vi "ObjectHandler.GetSegmentRefsForCycle.vi"(8 "error in (no error)":errorcluster, 10 "CycleName":string, 11 "ObjectHandler in":refnum<class "ObjectHandler.lvclass">) -> (0 "error out":errorcluster, 2 "ObjectArray":T1[](array[typedef]), 3 "ObjectHandler out":refnum<class "ObjectHandler.lvclass">)   [LabVIEW 2016, in "ObjectHandler.lvclass"]
uses:
  ObjectHandler.lvclass
  ObjectHandler.ObjectWType.ctl
  ObjectHandler.ObjectType.ctl
  ObjectHandler.lvclass/ObjectHandler.ctl
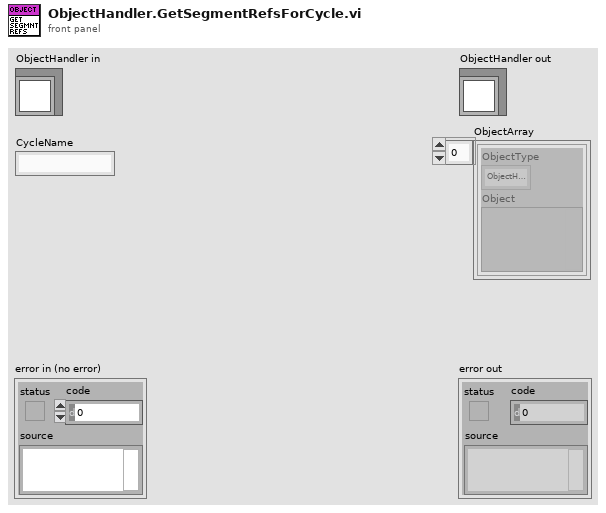
[diagram p1: front panel]
types:
  T1 = typedef "ObjectHandler.lvclass/ObjectHandler.ObjectWType.ctl" = cluster{"ObjectType":T2, "Object":variant}
  T2 = typedef "ObjectHandler.lvclass/ObjectHandler.ObjectType.ctl" = enum16{"undefined", "ObjectHandler", "ViHandler", "ErrorHandler", "CentralStorage", "Hausmodell", "Sondenmodell", "Wärmepumpe", "Umgebung"}
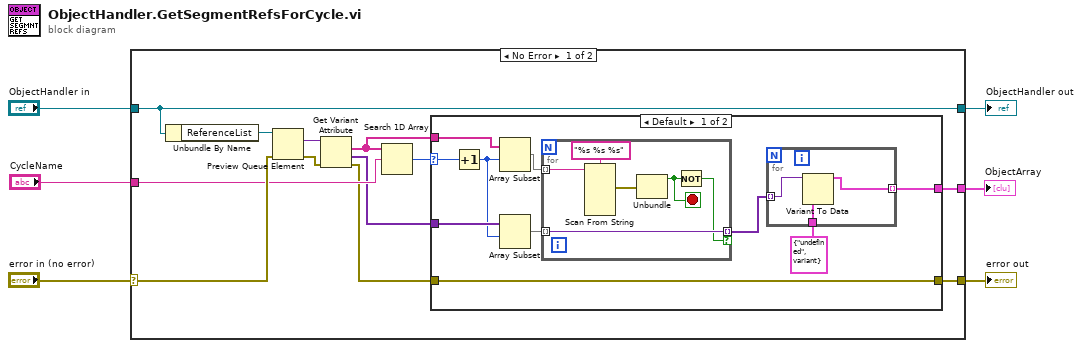
[diagram p0: block diagram]
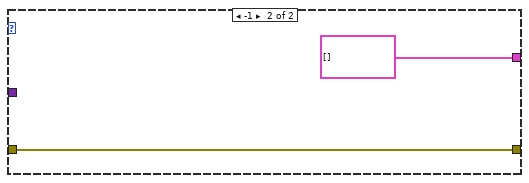
[diagram p2: hidden frame]
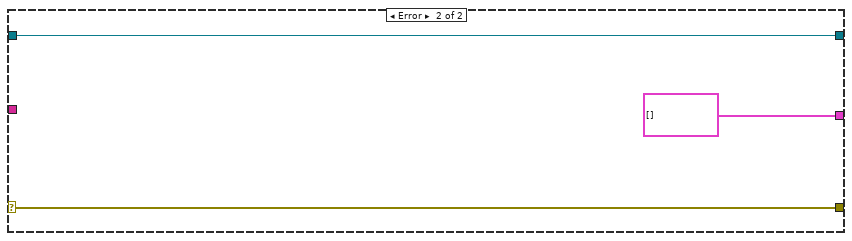
[diagram p3: hidden frame]
diagram:
  n1 = case shown="No Error" "error in (no error)" {
    selector: "error in (no error)" -> [w14 w42]
    tunnel: [w9 w42] -> w5
    tunnel: [w15 w41] -> w3
    tunnel: "ObjectHandler in" -> [w15 w41]
    tunnel: [w13 T1[] []] -> w2
    tunnel: "CycleName" -> [w12 _]
    frame No Error {
      n2 = Unbundle By Name(w15) -> ("ReferenceList"=w18:refnum<queue>)
      n3 = Preview Queue Element(queue=w18, error in (no error)=w14) -> (element=w17:variant, error out=w16:errorcluster)  [unwired: 1 in, 2 out]
      n4 = Get Variant Attribute(Variant=w17, error in=w16) -> (names=w7:string[], values=w8:variant[], error out=w10:errorcluster)  [unwired: 2 in, 1 out]
      n5 = Search 1D Array(1D array=w7, element=w12) -> (index of element=w11:i32)  [unwired: 1 in]
      n6 = case shown="Default" w11 {
        selector: w11 -> [w24 _]
        tunnel: [w27 T1[] []] -> w13
        tunnel: w10 -> [w26 w38]
        tunnel: [w26 w38] -> w9
        tunnel: w8 -> [w22 _]
        tunnel: w7 -> [w23 _]
        frame Default {
          n7 = Increment(x=w24) -> (x+1=w21:i32)
          n8 = Array Subset(array=w23, index=w21) -> (w25:string[])  [unwired: 1 in]
          n9 = Array Subset(array=w22, index=w21) -> (w20:variant[])  [unwired: 1 in]
          n10 = for {
            tunnel: w25 -> [w33] mode=indexing
            tunnel: w20 -> [w30] mode=indexing
            tunnel: [w30] -> w19 mode=indexing if=w29
            stop <- w31 stop-if-true
            n11 = Scan From String(format string="%s %s %s", input string=w33) -> (error out=w32:errorcluster)  [unwired: 8 in, 2 out]
            n12 = Unbundle(w32) -> ("status"=w31:bool)  [unwired: 2 out]
            n13 = Not(x=w31) -> (.not. x?=w29:bool)
          }
          n14 = for {
            tunnel: w19 -> [w37] mode=indexing
            tunnel: T1 {"ObjectType"=enum."undefined", "Object"=variant} ("ObjectWType") -> [w36]
            tunnel: [w35] -> w27 mode=indexing
            n15 = Variant To Data(type=w36, Variant=w37) -> (data=w35:T1)  [unwired: 1 in, 1 out]
          }
        }
        frame -1 {
        }
      }
    }
    frame Error {
    }
  }
  "error out" <- w5
  "ObjectHandler out" <- w3
  "ObjectArray" <- w2
